vi "Create From Variant (Object).vi"(8 "error in (no error)":errorcluster, 10 "Variant":variant, 11 "JSON Value in":refnum<class "JSON Value.lvclass">) -> (0 "error out":errorcluster, 3 "JSON Value out":refnum<class "JSON Value.lvclass">)   [LabVIEW 2016, in "JSON Value.lvclass"]
doc: "Creates a new JSON instance from the given Variant."
uses:
  JSON Helper/JSON Value.lvclass
  Insert Value (Multi).vi
  JSON String/New JSON String.vi
  <vilib>/Utility/Data Type/NI_Data Type.lvlib
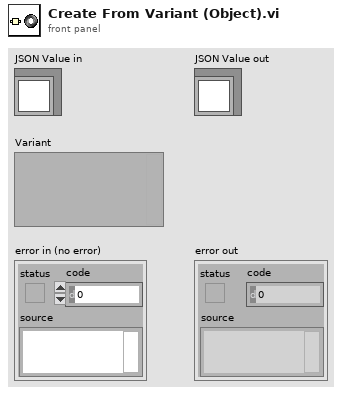
[diagram p1: front panel]
types:
  T1 = typedef "NI_Data Type.lvlib/Data Type.ctl" = enum8{"Invalid Type", "Void", "I8", "I16", "I32", "I64", "U8", "U16", "U32", "U64", "Single Float", "Double Float", "Extended Float", "Single Complex", "Double Complex", "Extended Complex", "Enum U8", "Enum U16", "Enum U32", "Enum U64", "Single Float With Unit", "Double Float With Unit", "Extended Float With Unit", "Single Complex with Unit", "Double Complex with Unit", "Extended Complex with Unit", "Boolean", "String", "Path", "Picture", "Tag", "Array", "Cluster", "Variant", "LV Variant", "Waveform", "Timestamp", "Digital Waveform", "Digital Data", "ExpressData", "Refnum", "External Data", "VI", "Poly VI", "LabVIEW Class Instance", "Fixed Point"}
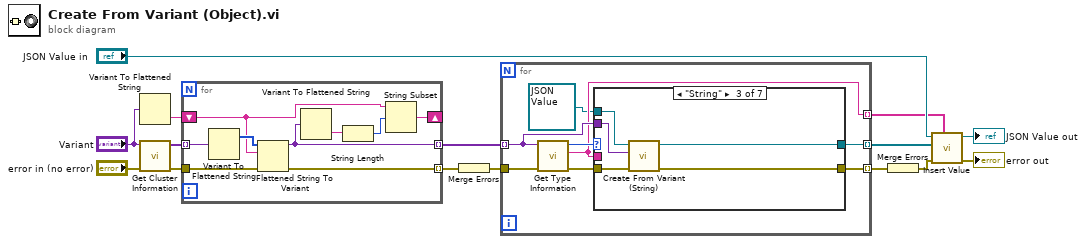
[diagram p0: block diagram]
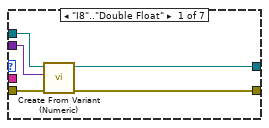
[diagram p2: hidden frame]
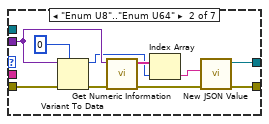
[diagram p3: hidden frame]
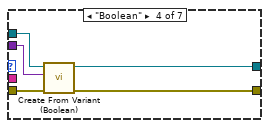
[diagram p4: hidden frame]
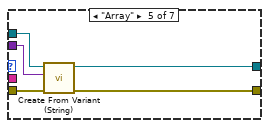
[diagram p5: hidden frame]
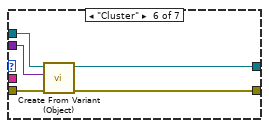
[diagram p6: hidden frame]
diagram:
  n1 = Variant To Flattened String(Variant="Variant") -> (data string=w15:string)  [unwired: 1 out]
  n2 = call <vilib>:"Get Cluster Information.vi"("error in (no error)"="error in (no error)", "Variant"="Variant") -> ("error out"=w12:errorcluster, "Cluster Elements"=w14:variant[])  [unwired: 8 in]
  n3 = for {
    tunnel: w14 -> [w24] mode=indexing
    tunnel: [w22] -> w13 mode=indexing
    shift-right: [w18] -> _
    shift-left: w15 -> [w21]
    tunnel: w12 -> [w17]
    tunnel: [w16] -> w11 mode=indexing
    n4 = Variant To Flattened String(Variant=w24) -> (1:w23:i16[])  [unwired: 1 out]
    n5 = Flattened String To Variant(4:w17, 6:w21, 7:w23) -> (0:w16:errorcluster, 3:w22:variant)
    n6 = Variant To Flattened String(Variant=w22) -> (data string=w20:string)  [unwired: 1 out]
    n7 = String Length(string=w20) -> (length=w19:i32)
    n8 = String Subset(string=w21, offset (0)=w19) -> (substring=w18:string)  [unwired: 1 in]
  }
  n9 = Merge Errors(w11) -> (w10:errorcluster)
  n10 = for {
    tunnel: w13 -> [w31] mode=indexing
    tunnel: [w30] -> w1 mode=indexing
    tunnel: [w29] -> w2 mode=indexing
    tunnel: w10 -> [w28]
    tunnel: [w26] -> w9 mode=indexing
    n11 = call <vilib>:"Get Type Information.vi"("error in (no error)"=w28, "Variant"=w31) -> ("error out"=w27:errorcluster, "Name"=w29:string, "Type"=w32:T1)  [unwired: 5 in, 2 out]
    n12 = case shown="\"String\"" w32 {
      tunnel: w31 -> [w37 w45 w52 w57 w62 w67 _]
      tunnel: [w34 w47 w49 w54 w61 w64 w68] -> w30
      tunnel: w29 -> [_ _ _ _ _ _ _]
      tunnel: w27 -> [w36 w40 w51 w56 w60 w66 w69]
      tunnel: [w35 w46 w50 w55 w59 w65 w69] -> w26
      tunnel: refnum<class "JSON Value.lvclass"> refnum ("JSON Object in") -> [w33 _ w48 w53 w58 w63 w68]
      frame "I8".."Double Float" {
        n13 = call "Create From Variant (Numeric).vi"("error in (no error)"=w36, "Variant"=w37, "JSON Value in"=w33) -> ("error out"=w35:errorcluster, "JSON Value out"=w34:refnum<class "JSON Value.lvclass">)  [unwired: 7 in]
      }
      frame "Enum U8".."Enum U64" {
        n14 = Variant To Data(error in=w40, type=u64 0, Variant=w45) -> (data=w42:u64, error out=w39:errorcluster)
        n15 = call <vilib>:"Get Numeric Information.vi"("error in (no error)"=w39, "Variant"=w45) -> ("error out"=w38:errorcluster, "Enum Names"=w43:string[])  [unwired: 6 in, 2 out]
        n16 = Index Array(array=w43, index=w42) -> (element=w41:string)
        n17 = call-poly "New JSON Value.vi"("error in (no error)"=w38, "value"=w41) -> ("error out"=w46:errorcluster, "JSON Value out"=w47:refnum<class "JSON Value.lvclass">)  [unwired: 8 in]
      }
      frame "String" {
        n18 = call "Create From Variant (String).vi"("error in (no error)"=w51, "Variant"=w52, "JSON Value in"=w48) -> ("error out"=w50:errorcluster, "JSON Value out"=w49:refnum<class "JSON Value.lvclass">)  [unwired: 7 in]
      }
      frame "Boolean" {
        n19 = call "Create From Variant (Boolean).vi"("error in (no error)"=w56, "Variant"=w57, "JSON Value in"=w53) -> ("error out"=w55:errorcluster, "JSON Value out"=w54:refnum<class "JSON Value.lvclass">)  [unwired: 7 in]
      }
      frame "Array" {
        n20 = call "Create From Variant (String).vi"("error in (no error)"=w60, "Variant"=w62, "JSON Value in"=w58) -> ("error out"=w59:errorcluster, "JSON Value out"=w61:refnum<class "JSON Value.lvclass">)  [unwired: 7 in]
      }
      frame "Cluster" {
        n21 = call "Create From Variant (Object).vi"("error in (no error)"=w66, "Variant"=w67, "JSON Value in"=w63) -> ("error out"=w65:errorcluster, "JSON Value out"=w64:refnum<class "JSON Value.lvclass">)  [unwired: 7 in]
      }
      frame Default {
      }
    }
  }
  n22 = Merge Errors(w9) -> (w8:errorcluster)
  n23 = call-poly "Insert Value.vi"("keys"=w2, "error in (no error)"=w8, "values"=w1, "JSON Value in"="JSON Value in") -> ("error out"=→"error out":errorcluster, "JSON Value out"=→"JSON Value out":refnum<class "JSON Value.lvclass">)  [unwired: 5 in, 1 out]
